vi "Record Frame Crop.vi"(8 "error in (no error)":errorcluster, 10 "Starting frame number":u32, 11 "Frame Grabber Data In in":T1={"Camera Session"="", "Frame"=refnum, "AVI Refnum"=refnum, "Codecs"=[], "Frame number"=0, "Tracking File Refnum"=refnum, "Tick Count"=0, "Probe Object"=refnum, "Playback Probe Data"=[], "Rigid Body"={"Position"={"x (mm)"=0.0, "y (mm)"=0.0, "z (mm)"=0.0}, "Orientation"={"Pitch (rad)"=0.0, "Yaw (rad)"=0.0, "Roll (rad)"=0.0}, "Quaternion"={"qx"=0.0, "qy"=0.0, "qz"=0.0, "qw"=0.0}, "Tracked?"=FALSE}, "Total no frames playback"=0, "Video FPS"=0.0, "Camera connected?"=FALSE, "Scene"=refnum, "Cropped Frame"=refnum, "Tracker FPS"=0.0, "Crop ROI"=[], "Presentation Values"=[], "Elapsed time (ms)"=0, "Camera frames playback"=0, "Refnums"={"Live Refnum"=refnum, "Record Refnum"=refnum, "Recording Settings Refnum"=refnum, "Playback Refnum"=refnum, "Frame Slider Refnum"=refnum, "Pause Refnum"=refnum, "Home Refnum"=refnum, "Crop Refnum"=refnum, "Clear Crop Refnum"=refnum, "stop refnum"=refnum, "Playback Rate Refnum"=refnum, "Operator Settings Refnums"=refnum, "Presentation Refnum"=refnum, "Gestation Refnum"=refnum, "Connection Settings Refnum"=refnum, "Crop Time Frame Slider Refnum"=refnum}, "Dimensions"={"Probe Dimensions"={"Probe Width"=0.0, "Probe Depth"=1.0, "Probe Height"=0.0}, "Room Dimensions"={"Room Width"=0.0, "Room Depth"=0.0, "Room Height"=0.0}}, "Playback Data As Strings"=[], "Cropped Tracking File Refnum"=refnum, "Cropped AVI Refnum"=refnum, "Header"=[]}) -> (0 "error out":errorcluster, 3 "Frame Grabber Data out":T1={"Camera Session"="", "Frame"=refnum, "AVI Refnum"=refnum, "Codecs"=[], "Frame number"=0, "Tracking File Refnum"=refnum, "Tick Count"=0, "Probe Object"=refnum, "Playback Probe Data"=[], "Rigid Body"={"Position"={"x (mm)"=0.0, "y (mm)"=0.0, "z (mm)"=0.0}, "Orientation"={"Pitch (rad)"=0.0, "Yaw (rad)"=0.0, "Roll (rad)"=0.0}, "Quaternion"={"qx"=0.0, "qy"=0.0, "qz"=0.0, "qw"=0.0}, "Tracked?"=FALSE}, "Total no frames playback"=0, "Video FPS"=0.0, "Camera connected?"=FALSE, "Scene"=refnum, "Cropped Frame"=refnum, "Tracker FPS"=0.0, "Crop ROI"=[], "Presentation Values"=[], "Elapsed time (ms)"=0, "Camera frames playback"=0, "Refnums"={"Live Refnum"=refnum, "Record Refnum"=refnum, "Recording Settings Refnum"=refnum, "Playback Refnum"=refnum, "Frame Slider Refnum"=refnum, "Pause Refnum"=refnum, "Home Refnum"=refnum, "Crop Refnum"=refnum, "Clear Crop Refnum"=refnum, "stop refnum"=refnum, "Playback Rate Refnum"=refnum, "Operator Settings Refnums"=refnum, "Presentation Refnum"=refnum, "Gestation Refnum"=refnum, "Connection Settings Refnum"=refnum, "Crop Time Frame Slider Refnum"=refnum}, "Dimensions"={"Probe Dimensions"={"Probe Width"=0.0, "Probe Depth"=1.0, "Probe Height"=0.0}, "Room Dimensions"={"Room Width"=0.0, "Room Depth"=0.0, "Room Height"=0.0}}, "Playback Data As Strings"=[], "Cropped Tracking File Refnum"=refnum, "Cropped AVI Refnum"=refnum, "Header"=[]})   [LabVIEW 2017]
uses:
  Controls/Frame Grabber Data.ctl
  <vilib>/userdefined/High Color/IMAQdx.ctl
  <vilib>/vision/Image Controls.llb/IMAQ Image.ctl
  <vilib>/vision/Avi.llb/IMAQ AVI2 Refnum.ctl
  Controls/Rigid Body Info.ctl
  Controls/Position.ctl
  Controls/Orientation.ctl
  Controls/Refnums.ctl
  Controls/Recording Settings.ctl
  Controls/Operator Settings.ctl
  Controls/Operator.ctl
  Controls/Dimensions.ctl
  Controls/Room Dimensions.ctl
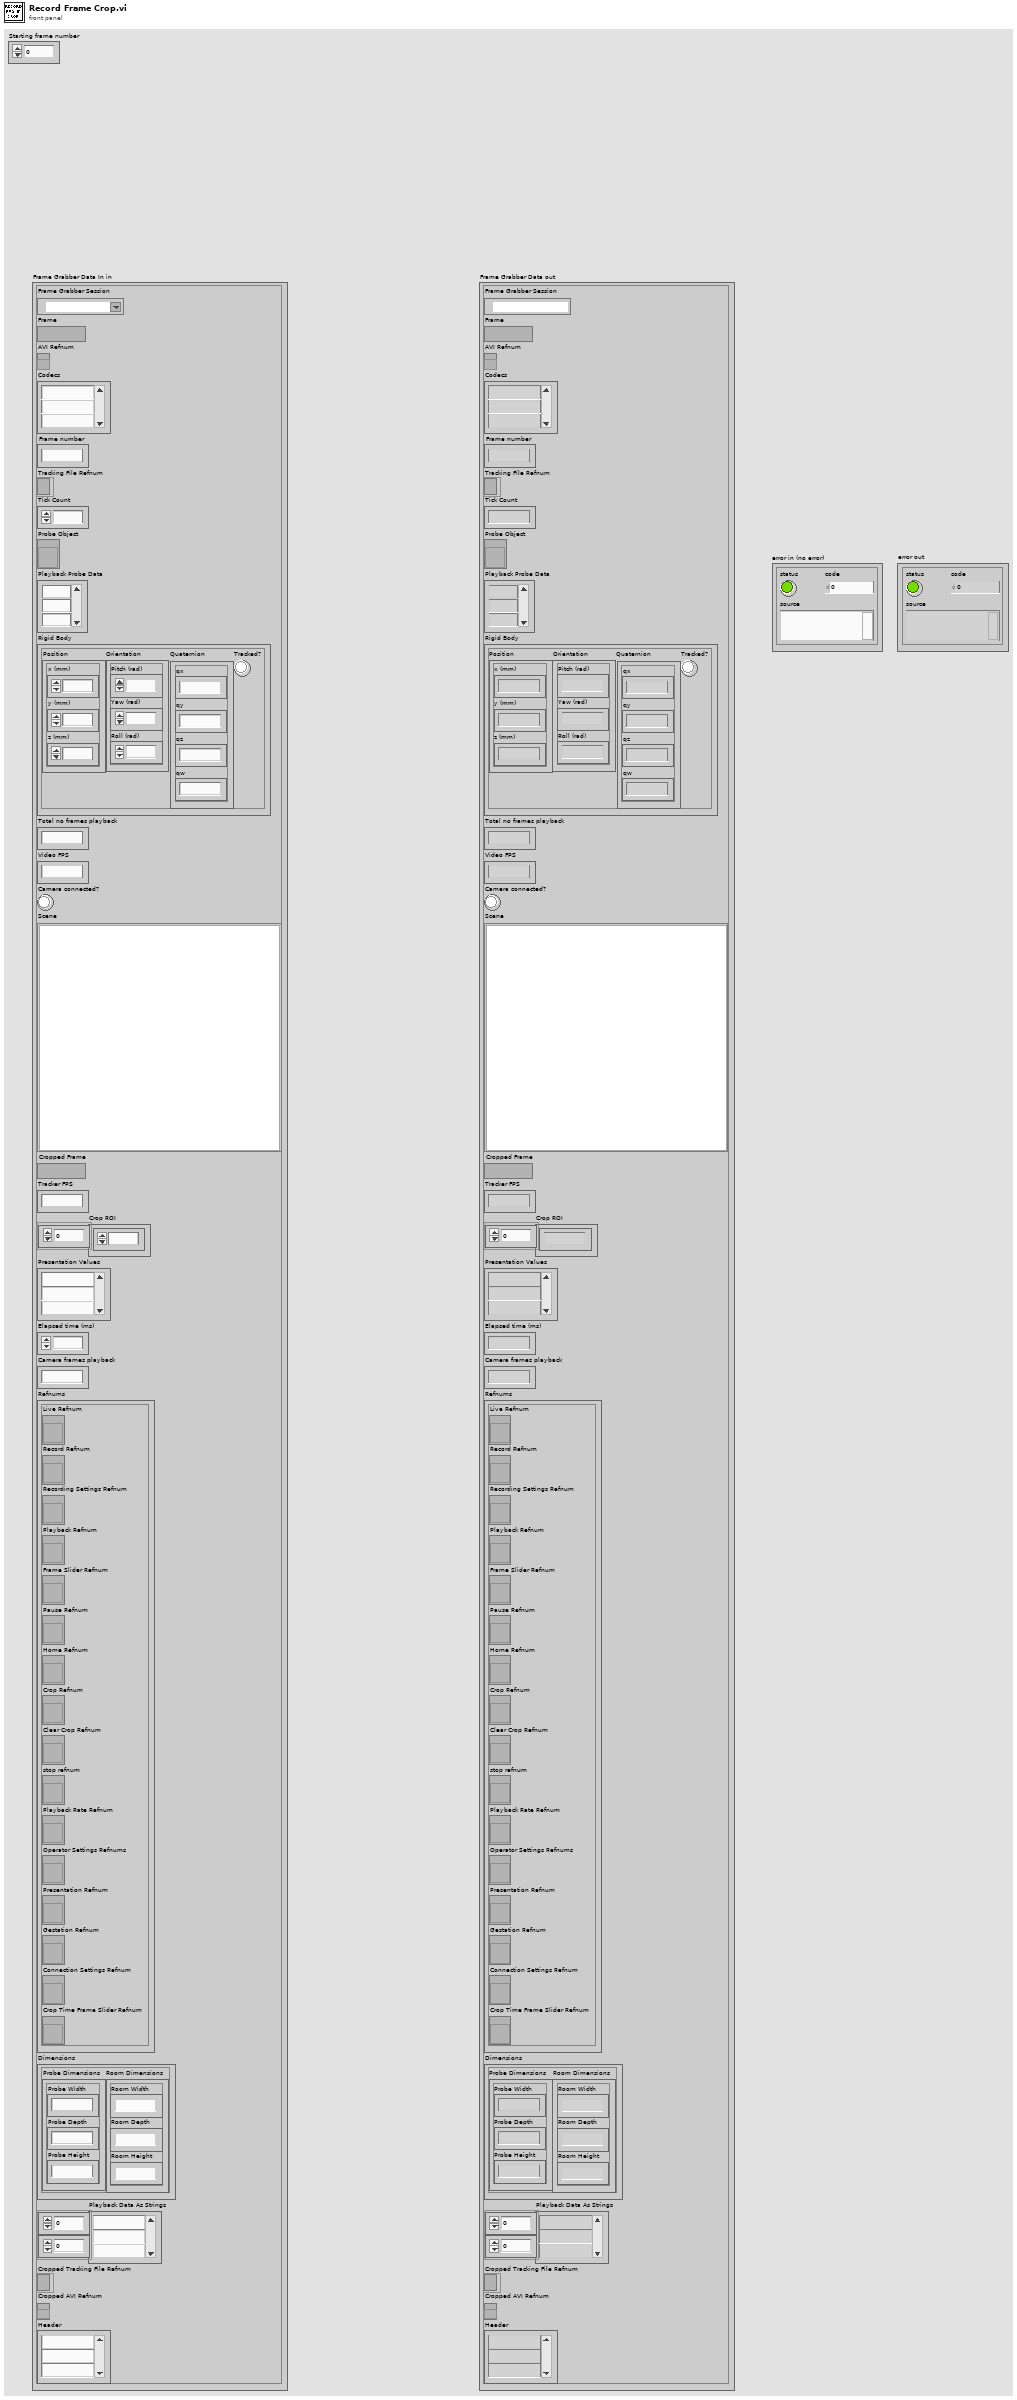
[diagram p1: front panel]
types:
  T1 = typedef "Frame Grabber Data.ctl" = cluster{"Camera Session":T2, "Frame":T3, "AVI Refnum":T4, "Codecs":string[], "Frame number":u32, "Tracking File Refnum":refnum<file>, "Tick Count":u32, "Probe Object":refnum<vi>, "Playback Probe Data":dbl[][], "Rigid Body":T5, "Total no frames playback":i32, "Video FPS":dbl, "Camera connected?":bool, "Scene":refnum<vi>, "Cropped Frame":T3, "Tracker FPS":dbl, "Crop ROI":i32[], "Presentation Values":string[], "Elapsed time (ms)":u32, "Camera frames playback":u32, "Refnums":T8, "Dimensions":T9, "Playback Data As Strings":string[][], "Cropped Tracking File Refnum":refnum<file>, "Cropped AVI Refnum":T4, "Header":string[]}
  T2 = typedef "IMAQdx.ctl" = refnum<k21>
  T3 = typedef "IMAQ Image.ctl" = refnum<image>
  T4 = typedef "IMAQ AVI2 Refnum.ctl" = refnum<k20>
  T5 = typedef "Rigid Body Info.ctl" = cluster{"Position":T6, "Orientation":T7, "Quaternion":cluster{"qx":sgl, "qy":sgl, "qz":sgl, "qw":sgl}, "Tracked?":bool}
  T6 = typedef "Position.ctl" = cluster{"x (mm)":sgl, "y (mm)":sgl, "z (mm)":sgl}
  T7 = typedef "Orientation.ctl" = cluster{"Pitch (rad)":sgl, "Yaw (rad)":sgl, "Roll (rad)":sgl}
  T8 = typedef "Refnums.ctl" = cluster{"Live Refnum":refnum<vi>, "Record Refnum":refnum<vi>, "Recording Settings Refnum":refnum<vi>, "Playback Refnum":refnum<vi>, "Frame Slider Refnum":refnum<vi>, "Pause Refnum":refnum<vi>, "Home Refnum":refnum<vi>, "Crop Refnum":refnum<vi>, "Clear Crop Refnum":refnum<vi>, "stop refnum":refnum<vi>, "Playback Rate Refnum":refnum<vi>, "Operator Settings Refnums":refnum<vi>, "Presentation Refnum":refnum<vi>, "Gestation Refnum":refnum<vi>, "Connection Settings Refnum":refnum<vi>, "Crop Time Frame Slider Refnum":refnum<vi>}
  T9 = typedef "Dimensions.ctl" = cluster{"Probe Dimensions":cluster{"Probe Width":sgl, "Probe Depth":sgl, "Probe Height":sgl}, "Room Dimensions":T10}
  T10 = typedef "Room Dimensions.ctl" = cluster{"Room Width":dbl, "Room Depth":dbl, "Room Height":dbl}
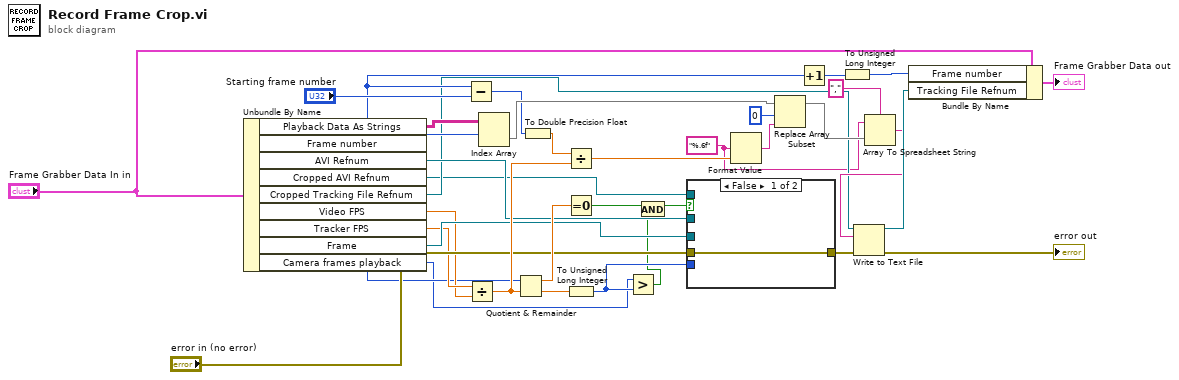
[diagram p0: block diagram]
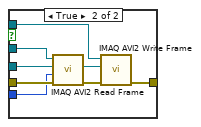
[diagram p2: hidden frame]
diagram:
  w5 = "%.6f" ("format string")
  n1 = Unbundle By Name("Frame Grabber Data In in") -> ("Playback Data As Strings"=w18:string[][], "Frame number"=w12:u32, "AVI Refnum"=w23:T4, "Cropped AVI Refnum"=w6:T4, "Cropped Tracking File Refnum"=w7:refnum<file>, "Video FPS"=w20:dbl, "Tracker FPS"=w21:dbl, "Frame"=w24:T3, "Camera frames playback"=w2:u32)
  n2 = Subtract(x=w12, y="Starting frame number") -> (x-y=w13:u32)
  n3 = Divide(x=w21, y=w20) -> (x/y=w30:dbl)
  n4 = Index Array(array=w18, index (row)=w12) -> (element=w17:string[])  [unwired: 1 in]
  n5 = Quotient & Remainder(x=w12, y=w30) -> (x-y*floor(x/y)=w31:dbl, floor(x/y)=w25:dbl)
  n6 = To Double Precision Float(number=w13) -> (double precision float=w28:dbl)
  n7 = Divide(x=w28, y=w30) -> (x/y=w27:dbl)
  n8 = Equal To 0?(x=w31) -> (x = 0?=w26:bool)
  n9 = To Unsigned Long Integer(number=w25) -> (unsigned 32bit integer=w3:u32)
  n10 = Greater?(x=w2, y=w3) -> (0:w1:bool)
  n11 = And(x=w26, y=w1) -> (x .and. y?=w4:bool)
  n12 = case shown="False" w4 {
    tunnel: [w36 w44] -> w35
    tunnel: "error in (no error)" -> [w36 w43]
    tunnel: w24 -> [_ w42]
    tunnel: w23 -> [_ w41]
    tunnel: w3 -> [_ w38]
    tunnel: w6 -> [_ w37]
    frame False {
    }
    frame True {
      n13 = call "IMAQ AVI2 Read Frame"("error in (no error)"=w43, "Frame Number"=w38, "Image"=w42, "AVI Refnum"=w41) -> ("error out"=w39:errorcluster, "Image Out"=w40:T3)  [unwired: 5 in, 1 out]
      n14 = call "IMAQ AVI2 Write Frame"("error in (no error)"=w39, "Image"=w40, "AVI Refnum"=w37) -> ("error out"=w44:errorcluster)  [unwired: 6 in, 2 out]
    }
  }
  n15 = Format Value(format string=w5, value (0)=w27) -> (output string=w15:string)  [unwired: 1 in]
  n16 = Replace Array Subset(array=w17, new element=w15, index=0) -> (w10:string[])
  n17 = Increment(x=w12) -> (x+1=w32:u32)
  n18 = To Unsigned Long Integer(number=w32) -> (unsigned 32bit integer=w14:u32)
  n19 = Array To Spreadsheet String(delimiter (Tab)=",", array=w10, 3:w5) -> (spreadsheet string=w8:string)
  n20 = Write to Text File(file (use dialog)=w7, text=w8, error in=w35) -> (refnum out=w34:refnum<file>, error out=→"error out":errorcluster)  [unwired: 1 in, 1 out]
  n21 = Bundle By Name(cluster="Frame Grabber Data In in", "Frame number"=w14, "Tracking File Refnum"=w34) -> (→"Frame Grabber Data out":T1)
